vi "NewExcel.vi"() -> (0 "error out":errorcluster, 3 "Excel out":refnum<class "Excel.lvclass">)   [LabVIEW 2015, in "Excel.lvclass"]
uses:
  Excel.lvclass
  Excel.lvclass/Excel.ctl
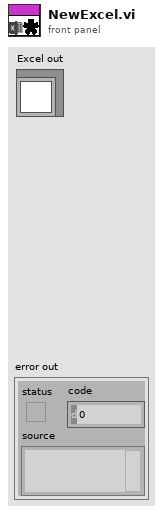
[diagram p1: front panel]
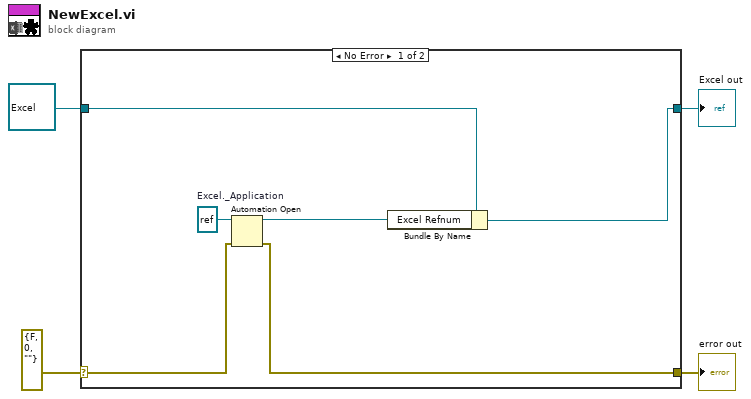
[diagram p0: block diagram]
diagram:
  n1 = case shown="No Error" errorcluster {"status"=FALSE, "code"=0, "source"=""} ("error in (no error)") {
    selector: errorcluster {"status"=FALSE, "code"=0, "source"=""} ("error in (no error)") -> [w9 w12]
    tunnel: [w8 w12] -> w3
    tunnel: [w5 w11] -> w1
    tunnel: refnum<class "Excel.lvclass"> refnum ("Excel in") -> [w7 w11]
    frame No Error {
      w10 = refnum<k7> refnum  # Excel._Application
      n2 = Automation Open(error in (no error)=w9, Automation Refnum=w10) -> (Automation Refnum=w6:refnum<k7>, error out=w8:errorcluster)  [unwired: 2 out]
      n3 = Bundle By Name(cluster=w7, "Excel Refnum"=w6) -> (w5:refnum<class "Excel.lvclass">)
    }
    frame Error {
    }
  }
  "error out" <- w3
  "Excel out" <- w1
